vi "test Import Bin File.vi"(8 "error in (no error)":errorcluster, 11 "TestCase in":refnum<class "AIM ARINC 664 Import.lvclass">) -> (0 "error out":errorcluster, 3 "TestCase out":refnum<class "AIM ARINC 664 Import.lvclass">)   [LabVIEW 2020, in "AIM ARINC 664 Import.lvclass"]
uses:
  AIM ARINC 664 Import.lvclass
  Scripting/AIM ARINC 664 Scripting.lvlib
  <userlib>/_OpenG.lib/appcontrol/appcontrol.llb/openg_application_control.lvlib
  <vilib>/NI/VeriStand Custom Device Testing Tools/VeriStandTestUtilities/VeriStandTestUtilities.lvlib
  <vilib>/addons/_JKI Toolkits/VI Tester/TestCase.llb/TestCase.lvclass
  C:/Program Files/National Instruments/LabVIEW 2024/vi.lib/addons/_JKI Toolkits/VI Tester/TestCase.llb/TestCase.lvclass
panel:
  out "Pass?":bool
  out "Expected failed (old bin)":cluster{path, bool}[](array[cluster])
  out "Expected to pass (new bin)":cluster{path, bool}[](array[cluster])
  out "Expected Errors":errorcluster[](array[cluster])
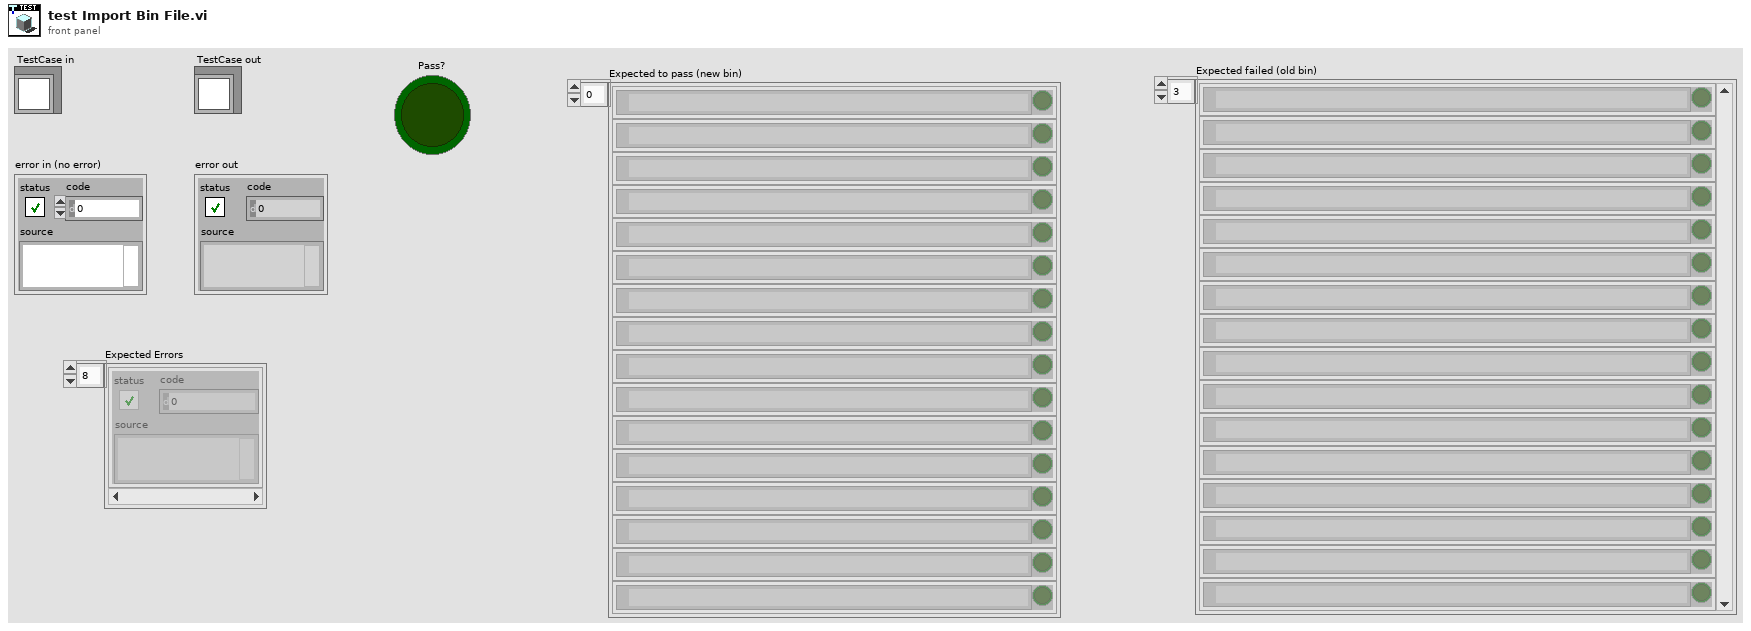
[diagram p1: front panel]
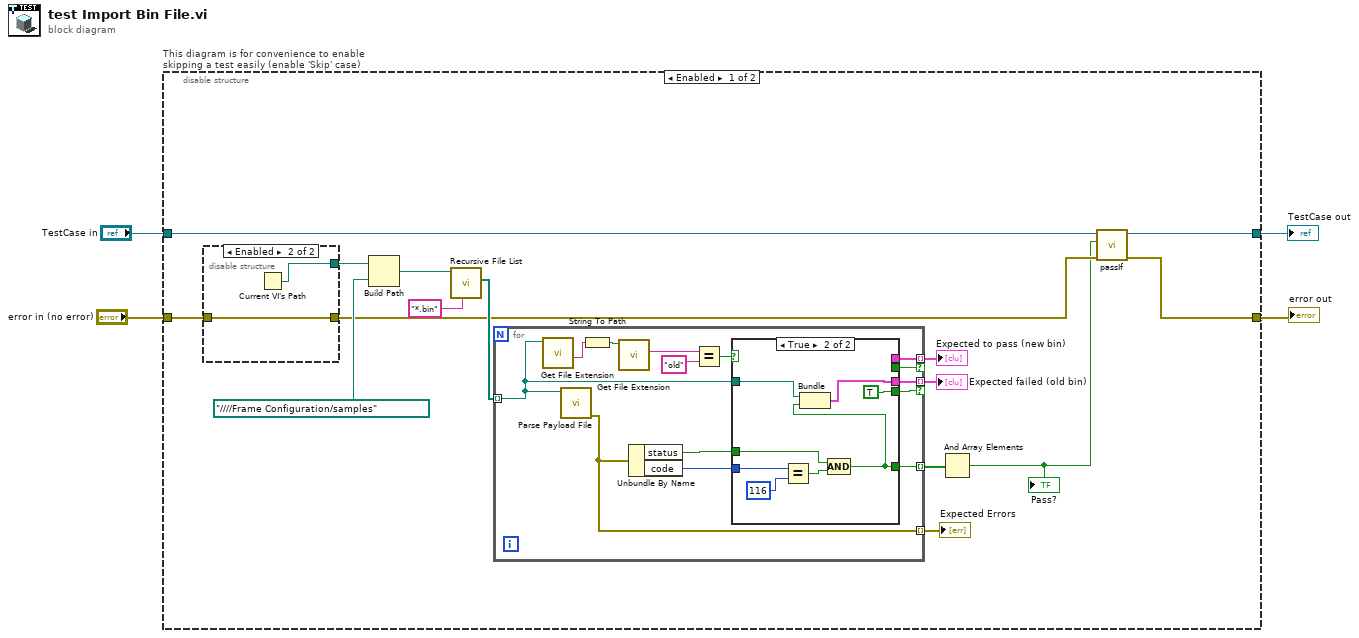
[diagram p0: block diagram]
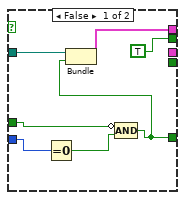
[diagram p2: hidden frame]
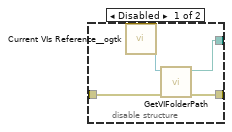
[diagram p3: hidden frame]
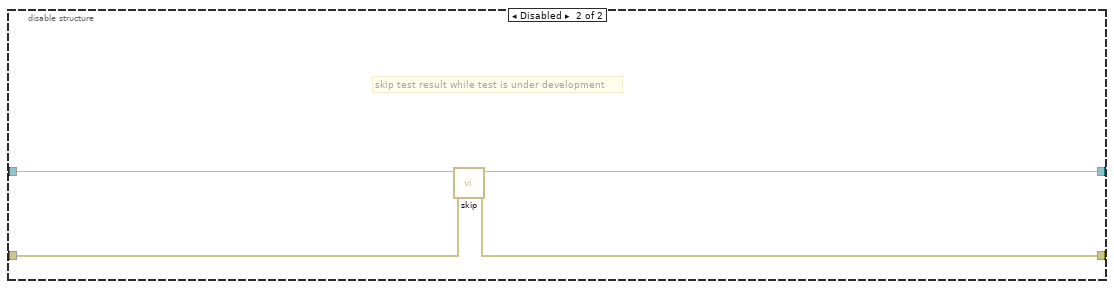
[diagram p4: hidden frame]
diagram:
  n1 = disable-structure "This diagram is for convenience to enable skipping a test easily (enable 'Skip' case)" shown="Enabled" {
    disable-tunnel: "TestCase in" -> [w11 w58]
    disable-tunnel: [w16 w56] -> w1
    disable-tunnel: [w15 w57] -> w3
    disable-tunnel: "error in (no error)" -> [w18 w55]
    frame Enabled {
      n2 = disable-structure shown="Enabled" {
        disable-tunnel: [w51 w54] -> w19
        disable-tunnel: w18 -> [w50 w53]
        disable-tunnel: [w49 w53] -> w10
        frame Disabled {
          n3 = call <userlib>:"Current VIs Reference__ogtk.vi"() -> ("Current VI's reference"=w52:refnum<vi>)  [unwired: 5 in]
          n4 = call <vilib>:"GetVIFolderPath.vi"("error in (no error)"=w50, "VI Reference in"=w52) -> ("error out"=w49:errorcluster, "VI Folder Path out"=w51:path)  [unwired: 8 in]
        }
        frame Enabled {
          n5 = Current VI's Path() -> (path=w54:path)
        }
      }
      n6 = Build Path(base path=w19, name or relative path=path "../../../../Frame Configuration/samples") -> (appended path=w9:path)
      n7 = call <vilib>:"Recursive File List.vi"("pattern"="*.bin", "Folder Path"=w9) -> ("All Files in Dir"=w13:path[])  [unwired: 5 in, 4 out]
      n8 = for {
        tunnel: w13 -> [w24] mode=indexing
        tunnel: [w29] -> w12 mode=indexing
        tunnel: [w23] -> w5 mode=indexing if=w22
        tunnel: [w25] -> w8 mode=indexing
        tunnel: [w21] -> w6 mode=indexing if=w20
        n9 = call <vilib>:"Get File Extension.vi"("file"=w24) -> ("filename without extension"=w33:string)  [unwired: 6 in, 4 out]
        n10 = call "Parse Payload File.vi"("frame array path in"=w24) -> ("error out"=w29:errorcluster)  [unwired: 8 in, 2 out]
        n11 = String To Path(string=w33) -> (path=w32:path)
        n12 = call <vilib>:"Get File Extension.vi"("file"=w32) -> ("lowercase file extension"=w31:string)  [unwired: 6 in, 4 out]
        n13 = Unbundle By Name(w29) -> ("status"=w27:bool, "code"=w26:i32)
        n14 = Equal?(x=w31, y="old") -> (x = y?=w28:bool)
        n15 = case shown="True" w28 {
          tunnel: w27 -> [w40 w46]
          tunnel: w26 -> [w39 w45]
          tunnel: [w34 w42] -> w25
          tunnel: w24 -> [w37 w43]
          tunnel: [_ w41] -> w23
          tunnel: [_ TRUE] -> w22
          tunnel: [w35 _] -> w21
          tunnel: [TRUE _] -> w20
          frame False {
            n16 = Equal To 0?(x=w39) -> (x = 0?=w38:bool)
            n17 = Compound Arithmetic op=AND(invert w40, w38) -> (w34:bool)
            n18 = Bundle(w37, w34) -> (w35:cluster{path, bool})  [unwired: 1 in]
          }
          frame True {
            n19 = Equal?(x=w45, y=116) -> (x = y?=w47:bool)
            n20 = Compound Arithmetic op=AND(w46, w47) -> (w42:bool)
            n21 = Bundle(w43, w42) -> (w41:cluster{path, bool})  [unwired: 1 in]
          }
        }
      }
      "Expected Errors" <- w12
      "Expected to pass (new bin)" <- w6
      "Expected failed (old bin)" <- w5
      n22 = And Array Elements(Boolean array=w8) -> (logical AND=w7:bool)
      "Pass?" <- w7
      n23 = call-dynamic "passIf.vi"("error in (no error)"=w10, "pass"=w7, "TestCase in"=w11) -> ("error out"=w15:errorcluster, "TestCase out"=w16:refnum<class "AIM ARINC 664 Import.lvclass">)  [unwired: 7 in]
    }
    frame Disabled {
      # "skip test result while test is under development"
      n24 = call <vilib>:"skip.vi"("error in (no error)"=w55, "TestCase in"=w58) -> ("error out"=w57:errorcluster, "TestCase out"=w56:refnum<class "AIM ARINC 664 Import.lvclass">)  [unwired: 8 in]
    }
  }
  "error out" <- w3
  "TestCase out" <- w1
